vi "Add_new_Columns_to_file_Low.vi"(0 "Filename":path, 5 "Merged Channels":string[](array[string]), 7 "String to add":string[][](array[string]), 9 "Start of data (bytes)":i32, 11 "Start of read offset (chars.: 0)":i32) -> ()   [LabVIEW 2010]
uses:
  Anemometry/Anemometry Sub Vis/Globals/Constants_global.vi
panel:
  in  "stop":bool
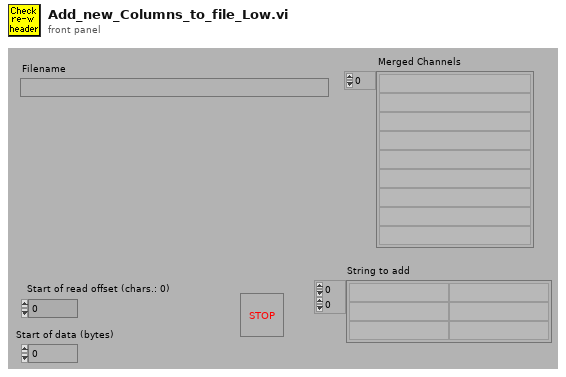
[diagram p1: front panel]
types:
  T1 = enum16{"read/write", "read-only", "write-only", "write-only (truncate)"}
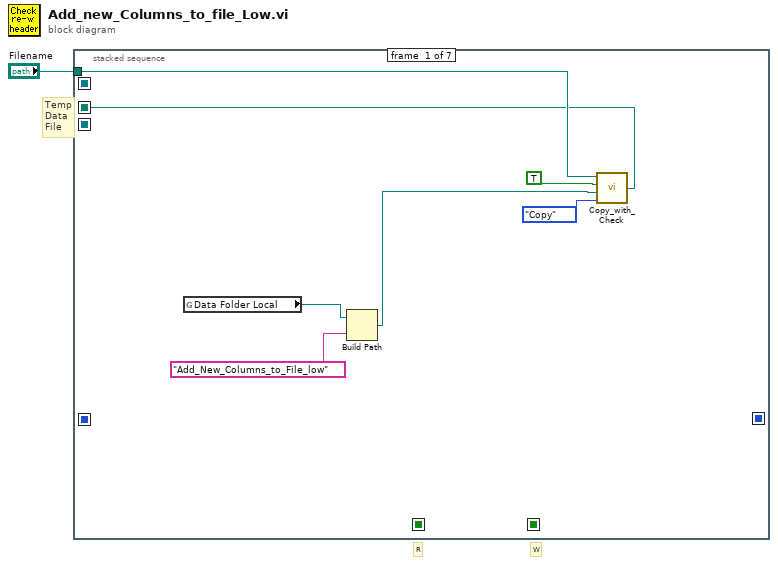
[diagram p0: block diagram]
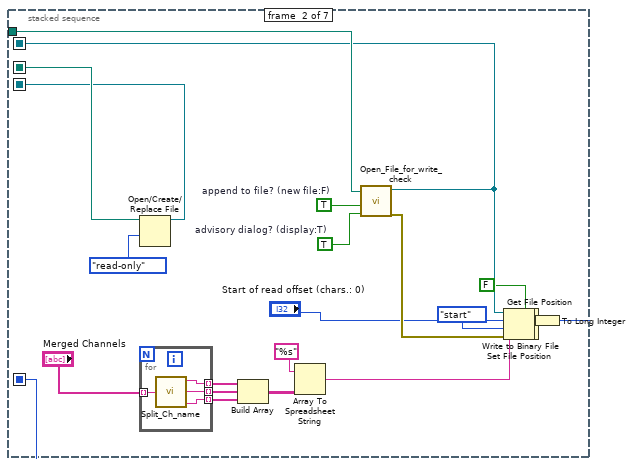
[diagram p2: hidden frame]
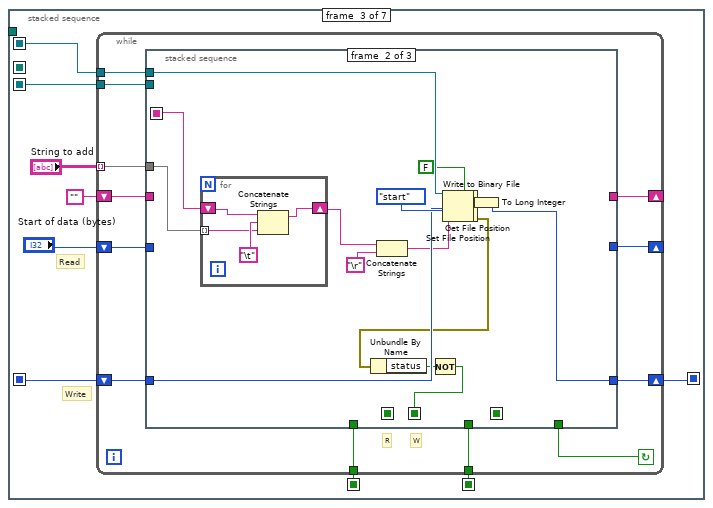
[diagram p3: hidden frame]
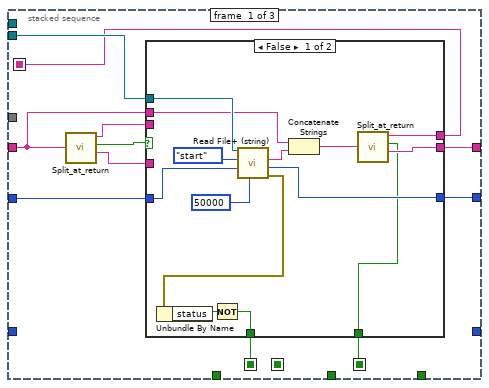
[diagram p4: hidden frame]
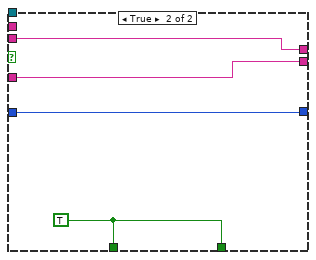
[diagram p5: hidden frame]
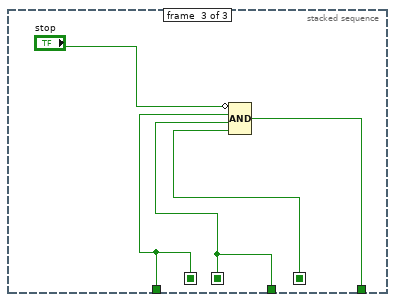
[diagram p6: hidden frame]
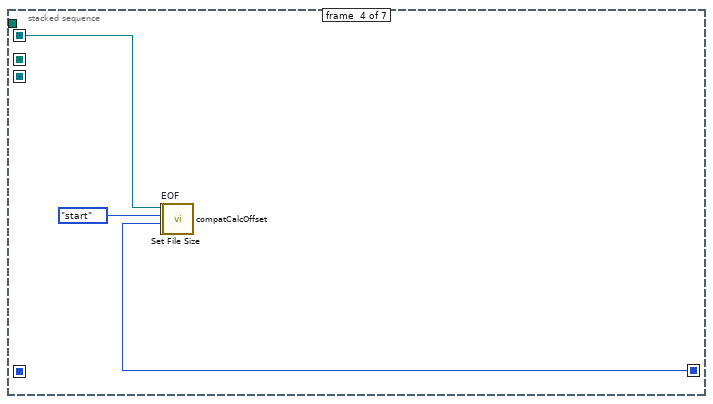
[diagram p7: hidden frame]
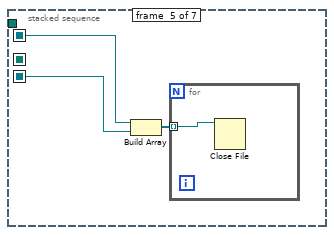
[diagram p8: hidden frame]
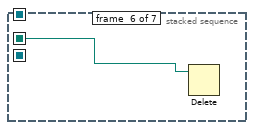
[diagram p9: hidden frame]
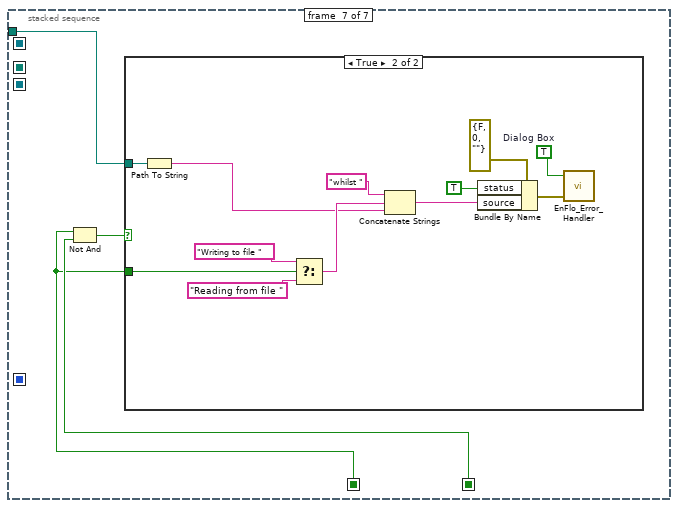
[diagram p10: hidden frame]
diagram:
  # "W"
  # "R"
  # "Temp\nData\nFile"
  n1 = stacked-sequence {
    seq-local: [w3 _ _ _ _ _ _] -> [_ w28 _ _ _ w124 _]
    seq-local: [_ w27 _ _ _ _ _] -> [_ _ w44 _ w121 _ _]
    seq-local: [_ w23 _ _ _ _ _] -> [_ _ w42 w119 w122 _ _]
    seq-local: [_ w15 _ _ _ _ _] -> [_ _ w43 _ _ _ _]
    seq-local: [_ _ w41 _ _ _ _] -> [_ _ _ _ _ _ w126]
    seq-local: [_ _ w40 _ _ _ _] -> [_ _ _ _ _ _ w128]
    seq-local: [_ _ w39 _ _ _ _] -> [_ _ _ w118 _ _ _]
    tunnel: "Filename" -> [w4 w29 _ _ _ _ w125]
    frame #0 {
      n2 = global read "Constants_global.vi" "Data Folder Local"() -> (w6:path)
      n3 = Build Path(base path=w6, name or relative path="Add_New_Columns_to_File_low") -> (appended path=w8:path)
      n4 = call "Copy_with_Check.vi"("Mode"=enum16{"Move", "Copy"}."Copy", "Target Path"=w8, "Variable Target?"=TRUE, "Source Path"=w4) -> ("Pathname Out"=w3:path)
    }
    frame #1 {
      w30 = TRUE  # advisory dialog? (display:T)
      w31 = TRUE  # append to file? (new file:F)
      n5 = Open/Create/Replace File(file path (use dialog)=w28, access (0:read/write)=T1."read-only" ("open mode (0)")) -> (refnum out=w27:refnum<file>)  [unwired: 1 in, 5 out]
      n6 = for {
        tunnel: "Merged Channels" -> [w36] mode=indexing
        tunnel: [w35] -> w26 mode=indexing
        tunnel: [w34] -> w25 mode=indexing
        tunnel: [w33] -> w24 mode=indexing
        n7 = call "Split_Ch_name.vi"("Ch name"=w36) -> ("Top level"=w35:string, "Middle"=w34:string, "Low level"=w33:string)
      }
      n8 = Build Array(w26, w25, w24) -> (w21:string[][])
      n9 = Array To Spreadsheet String(array=w21, 3:"%s" ("format string")) -> (spreadsheet string=w19:string)  [unwired: 1 out]
      n10 = call "Open_File_for_write_check.vi"("advisory dialog? (display:T)"=w30, "append to file? (new file:F)"=w31, "file path"=w29) -> ("error out"=w18:errorcluster, "refnum"=w23:refnum<file>)  [unwired: 7 out]
      n11 = Set File Position(offset (in bytes) (0)="Start of read offset (chars.: 0)", refnum=w23, from (0:start)=enum16{"start", "end", "current"}."start" ("pos mode (0:2)"), error in=w18) -> (refnum out=w14:refnum<file>, error out=w13:errorcluster)
      n12 = Write to Binary File(file (use dialog)=w14, data=w19, error in=w13, 5:FALSE ("prepend array or string size? (T)")) -> (refnum out=w12:refnum<file>, error out=w11:errorcluster)  [unwired: 3 out]
      n13 = Get File Position(4:w11, 7:w12) -> (2:w10:i64)  [unwired: 2 out]
      n14 = To Long Integer(number=w10) -> (32bit integer=w15:i32)
    }
    frame #2 {
      # "Write"
      # "Read"
      n15 = while {
        tunnel: "String to add" -> [w46] mode=indexing
        tunnel: [w48] -> w40
        tunnel: [w49] -> w41
        tunnel: w42 -> [w52]
        shift-left: w43 -> [w53]
        shift-right: [w51] -> w39
        tunnel: w44 -> [w55]
        shift-left: "Start of data (bytes)" -> [w57]
        shift-right: [w56] -> _
        shift-left: "" -> [w47]
        shift-right: [w54] -> _
        stop <- w50 continue-if-true
        # "R"
        # "W"
        n16 = stacked-sequence {
          seq-local: [w60 _ _] -> [_ w98 _]
          seq-local: [_ w99 _] -> [_ _ w109]
          seq-local: [w61 _ _] -> [_ _ w111]
          seq-local: [w62 _ _] -> [_ _ w110]
          tunnel: w47 -> [w65 _ _]
          tunnel: w57 -> [w68 _ _]
          tunnel: [w67 _ _] -> w56
          tunnel: w55 -> [w66 _ _]
          tunnel: [w64 _ _] -> w54
          tunnel: w53 -> [_ w103 _]
          tunnel: w52 -> [_ w102 _]
          tunnel: [_ w93 _] -> w51
          tunnel: [_ _ w112] -> w50
          tunnel: [_ _ w110] -> w49
          tunnel: [_ _ w109] -> w48
          tunnel: w46 -> [_ w97 _]
          frame #0 {
            n17 = call "Split_at_return.vi"("String"=w65) -> ("before substring"=w59:string, "Matched?"=w58:bool, "after substring"=w63:string)  [unwired: 1 in, 1 out]
            n18 = case shown="False" w58 {
              tunnel: w68 -> [w81 w86]
              tunnel: [w79 w86] -> w67
              tunnel: w66 -> [w78 _]
              tunnel: w65 -> [w76 _]
              tunnel: [w74 w85] -> w64
              tunnel: w63 -> [_ w85]
              tunnel: [w71 w84] -> w62
              tunnel: [w69 w84] -> w61
              tunnel: [w70 w83] -> w60
              tunnel: w59 -> [_ w83]
              frame False {
                n19 = call <vilib>:"Read File+ (string).vi"("count"=50000, "pos offset (bytes:0)"=w81, "pos mode (rel. to current:2)"=enum16{"start", "end", "current"}."start", "refnum"=w78) -> ("error out"=w73:errorcluster, "mark after read (bytes)"=w79:i32, "string"=w77:string)  [unwired: 1 in, 4 out]
                n20 = Unbundle By Name(w73) -> ("status"=w72:bool)
                n21 = Not(x=w72) -> (.not. x?=w71:bool)
                n22 = Concatenate Strings(w76, w77) -> (w75:string)
                n23 = call "Split_at_return.vi"("String"=w75) -> ("before substring"=w70:string, "Matched?"=w69:bool, "after substring"=w74:string)  [unwired: 1 in, 1 out]
              }
              frame True {
                w84 = TRUE
              }
            }
          }
          frame #1 {
            n24 = for {
              shift-right: [w107] -> w95
              shift-left: w98 -> [w108]
              tunnel: w97 -> [w105] mode=indexing
              n25 = Concatenate Strings(w108, "\t", w105) -> (w107:string)
            }
            n26 = Concatenate Strings(w95, "\r") -> (w96:string)
            n27 = Set File Position(offset (in bytes) (0)=w103, refnum=w102, from (0:start)=enum16{"start", "end", "current"}."start" ("pos mode (0:2)")) -> (refnum out=w92:refnum<file>, error out=w91:errorcluster)  [unwired: 1 in]
            n28 = Write to Binary File(file (use dialog)=w92, data=w96, error in=w91, 5:FALSE ("prepend array or string size? (T)")) -> (refnum out=w90:refnum<file>, error out=w89:errorcluster)  [unwired: 3 out]
            n29 = Get File Position(4:w89, 7:w90) -> (0:w101:errorcluster, 2:w88:i64)  [unwired: 1 out]
            n30 = Unbundle By Name(w101) -> ("status"=w100:bool)
            n31 = Not(x=w100) -> (.not. x?=w99:bool)
            n32 = To Long Integer(number=w88) -> (32bit integer=w93:i32)
          }
          frame #2 {
            n33 = Compound Arithmetic op=AND(invert "stop", w110, w109, w111) -> (w112:bool)
          }
        }
      }
    }
    frame #3 {
      n34 = call <vilib>:"compatCalcOffset.vi"("pos offset (0)"=w118, "pos mode (0:1)"=enum16{"start", "end", "current"}."start", "refnum"=w119) -> ("error out"=w116:errorcluster, "offset"=w115:i32, "dup refnum"=w114:refnum<file>)  [unwired: 1 in, 5 out]
      n35 = Set File Size "EOF"(4:w116, 6:w115, 7:w114) -> ()  [unwired: 2 out]
    }
    frame #4 {
      n36 = Build Array(w122, w121) -> (w120:refnum<file>[])
      n37 = for {
        tunnel: w120 -> [w123] mode=indexing
        n38 = Close File(refnum=w123) -> ()  [unwired: 1 in, 2 out]
      }
    }
    frame #5 {
      n39 = Delete(path (use dialog)=w124) -> ()  [unwired: 1 in, 6 out]
    }
    frame #6 {
      n40 = Not And(1:w128, 2:w126) -> (0:w127:bool)
      n41 = case shown="True" w127 {
        tunnel: w126 -> [_ w140]
        tunnel: w125 -> [_ w130]
        frame False {
        }
        frame True {
          w133 = TRUE  # Dialog Box
          n42 = Path To String(path=w130) -> (string=w129:string)
          n43 = Select(t="Writing to file ", s=w140, f="Reading from file ") -> (s? t:f=w136:string)
          n44 = Concatenate Strings("whilst ", w136, w129) -> (w131:string)
          n45 = Bundle By Name(cluster=errorcluster {"status"=FALSE, "code"=0, "source"=""} ("error in (no error)"), "status"=TRUE ("Bundle Element"), "source"=w131) -> (w134:errorcluster)
          n46 = call "EnFlo_Error_Handler.vi"("error in (no error)"=w134, "Dialog Box (T)"=w133) -> ()  [unwired: 1 in, 3 out]
        }
      }
    }
  }
